vi "DestroyPublicEvents.vi"(8 "error in (no error)":errorcluster, 11 "SMO":refnum<class "SMO.lvclass">) -> (0 "error out":errorcluster, 3 "SMO out":refnum<class "SMO.lvclass">)   [LabVIEW 2019, in "SMO.lvclass"]
doc: "JKI State Machine Objects (SMO) 1.3.0.56\nJKI - JKI\nCopyright (c) 2017, JKI"
uses:
  SMO.lvclass
panel:
  # "For instructions on how to use the JKI State Machine Objects, examples and video tutorials, visit:\nhttp://jki.net/state-machine-objects/\n\nJKI State Machine Objects™\nhttp://jki.net/state-machine-objects/\nCopyright (C) 2005-2015, JKI <info@jki.net>\nALL RIGHTS RESERVED"
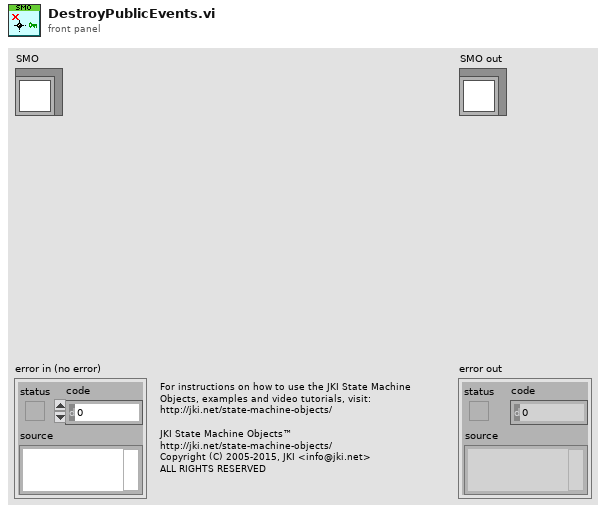
[diagram p1: front panel]
types:
  T1 = typedef "SMO.lvclass/Public Events.ctl" = cluster{"Error":refnum<user-event>, "State":refnum<user-event>, "Reserve State":refnum<user-event>}
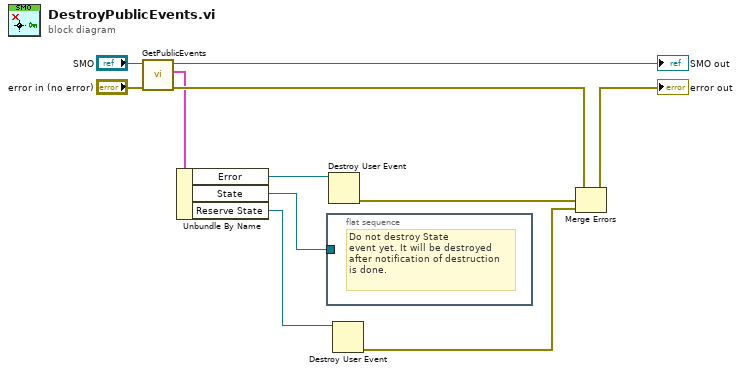
[diagram p0: block diagram]
diagram:
  n1 = call "GetPublicEvents.vi"("error in (no error)"="error in (no error)", "SMO"="SMO") -> ("error out"=w7:errorcluster, "Public Events"=w6:T1, "SMO out"=→"SMO out":refnum<class "SMO.lvclass">)  [unwired: 7 in]
  n2 = Unbundle By Name(w6) -> ("Error"=w5:refnum<user-event>, "State"=w3:refnum<user-event>, "Reserve State"=w2:refnum<user-event>)
  n3 = flat-sequence {
    tunnel: w3 -> [_]
    frame #0 {
      # "Do not destroy State\nevent yet. It will be destroyed\nafter notification of destruction\nis done."
    }
  }
  n4 = Destroy User Event(user event=w5) -> (error out=w4:errorcluster)  [unwired: 1 in]
  n5 = Destroy User Event(user event=w2) -> (error out=w1:errorcluster)  [unwired: 1 in]
  n6 = Merge Errors(w7, w4, w1) -> (→"error out":errorcluster)
